vi "Hardware XML Write (Ballard-1533).vi"(8 "error in":errorcluster, 11 "xml ref in":refnum<k24>) -> (0 "error out":errorcluster, 3 "xml ref out":refnum<k24>)   [LabVIEW 2020]
uses:
  C:/Users/Administrator/Desktop/GIT/Ballard-MIL-STD-1553-Custom-Device/Source/System Explorer/SubVIs/Parse XML Ballard/1.2/BTIXML_SerDes.dll
  Ballard-MIL-STD-1553-Custom-Device/Source/System Explorer/SubVIs/Parse XML Ballard/1.2/BTIXML_SerDes.dll
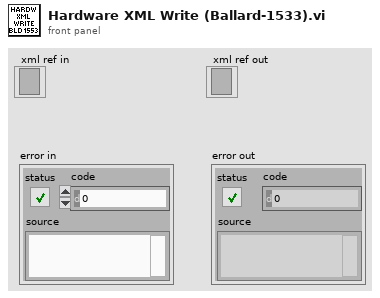
[diagram p1: front panel]
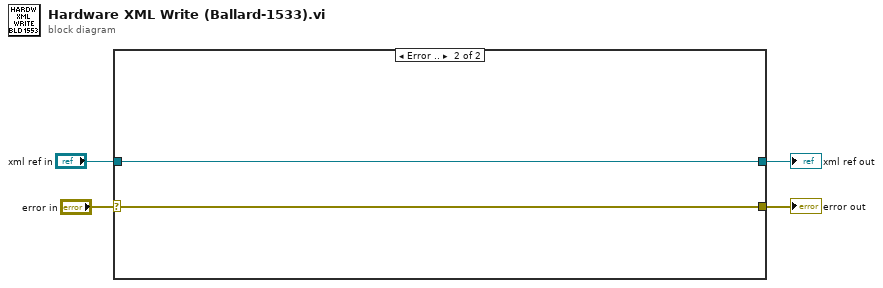
[diagram p0: block diagram]
diagram:
  n1 = case shown="Error .." "error in" {
    selector: "error in" -> [w5 w7]
    tunnel: "xml ref in" -> [w6 w8]
    tunnel: [w6 w8] -> w2
    tunnel: [w5 w7] -> w1
    frame No Error {
    }
    frame Error {
    }
  }
  "xml ref out" <- w2
  "error out" <- w1
